vi "PH_Synchrolock_Watch.establish connection.vi"(0 "i ref in":refnum<vi>, 5 "error in":errorcluster) -> (14 "i ref out":refnum<vi>, 19 "error out":errorcluster)   [LabVIEW 2014, in "PH_Synchrolock_Watch.lvlib"]
doc: "This VI checks the connection and resets the hardware."
uses:
  PH_Synchrolock_Watch.lvlib
  PH_TKTDS-30xx/PH_TKTDS-30xx.lvlib
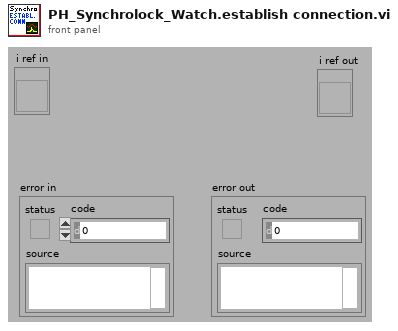
[diagram p1: front panel]
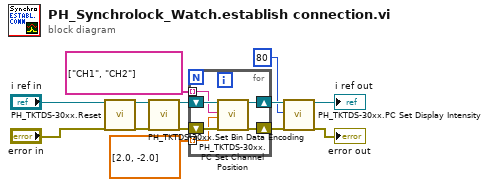
[diagram p0: block diagram]
diagram:
  n1 = call "PH_TKTDS-30xx.Reset.vi"("i ref in"="i ref in", "error IO"="error in") -> ("i ref out"=w12:refnum<vi>, "error out"=w10:errorcluster)  [unwired: 16 in]
  n2 = call "PH_TKTDS-30xx.Set Bin Data Encoding.vi"("i ref in"=w12, "error IO"=w10) -> ("i ref out"=w7:refnum<vi>, "error out"=w9:errorcluster)  [unwired: 16 in]
  n3 = for {
    shift-right: [w16] -> w4
    shift-left: w7 -> [w17]
    shift-right: [w18] -> w5
    shift-left: w9 -> [w19]
    tunnel: string[] ["CH1", "CH2"] -> [w15] mode=indexing
    tunnel: dbl[] [2.0, -2.0] -> [w14] mode=indexing
    n4 = call "PH_TKTDS-30xx.PC Set Channel Position.vi"("i ref in"=w17, "Channel Name"=w15, "Position (0)"=w14, "error IO"=w19) -> ("i ref out"=w16:refnum<vi>, "error out"=w18:errorcluster)  [unwired: 14 in]
  }
  n5 = call "PH_TKTDS-30xx.PC Set Display Intensity.vi"("i ref in"=w4, "Intensity (1)"=u8 80, "error IO"=w5) -> ("i ref out"=→"i ref out":refnum<vi>, "error out"=→"error out":errorcluster)  [unwired: 15 in]
